vi "子VI-计算分辨率后的值.vi"(7 "测量结果":dbl[][](array[numeric]), 9 "图像X向分辨率（mm/像素）":dbl, 10 "图像Y向分辨率（mm/像素）":dbl) -> (1 "初始化的数组":dbl[][](array[numeric]))   [LabVIEW 2018]
panel:
  out "测量结果 2":dbl[](array[numeric])
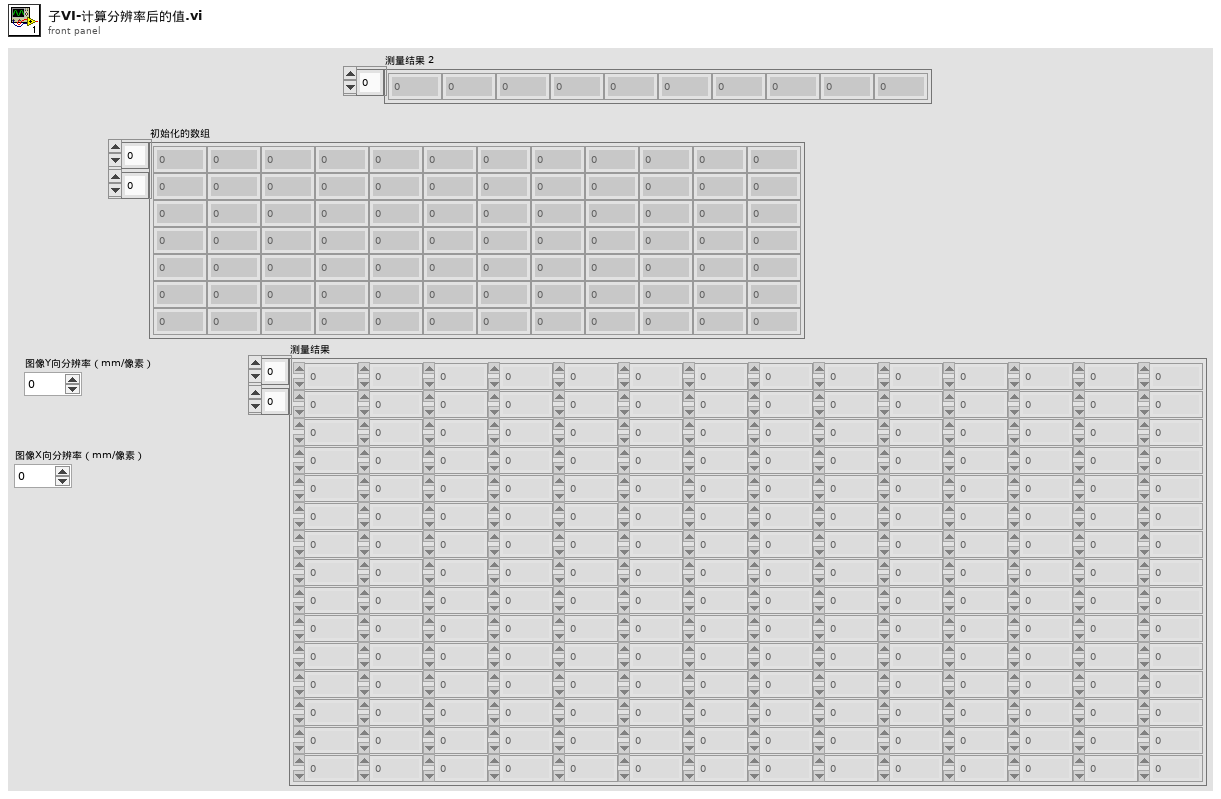
[diagram p1: front panel]
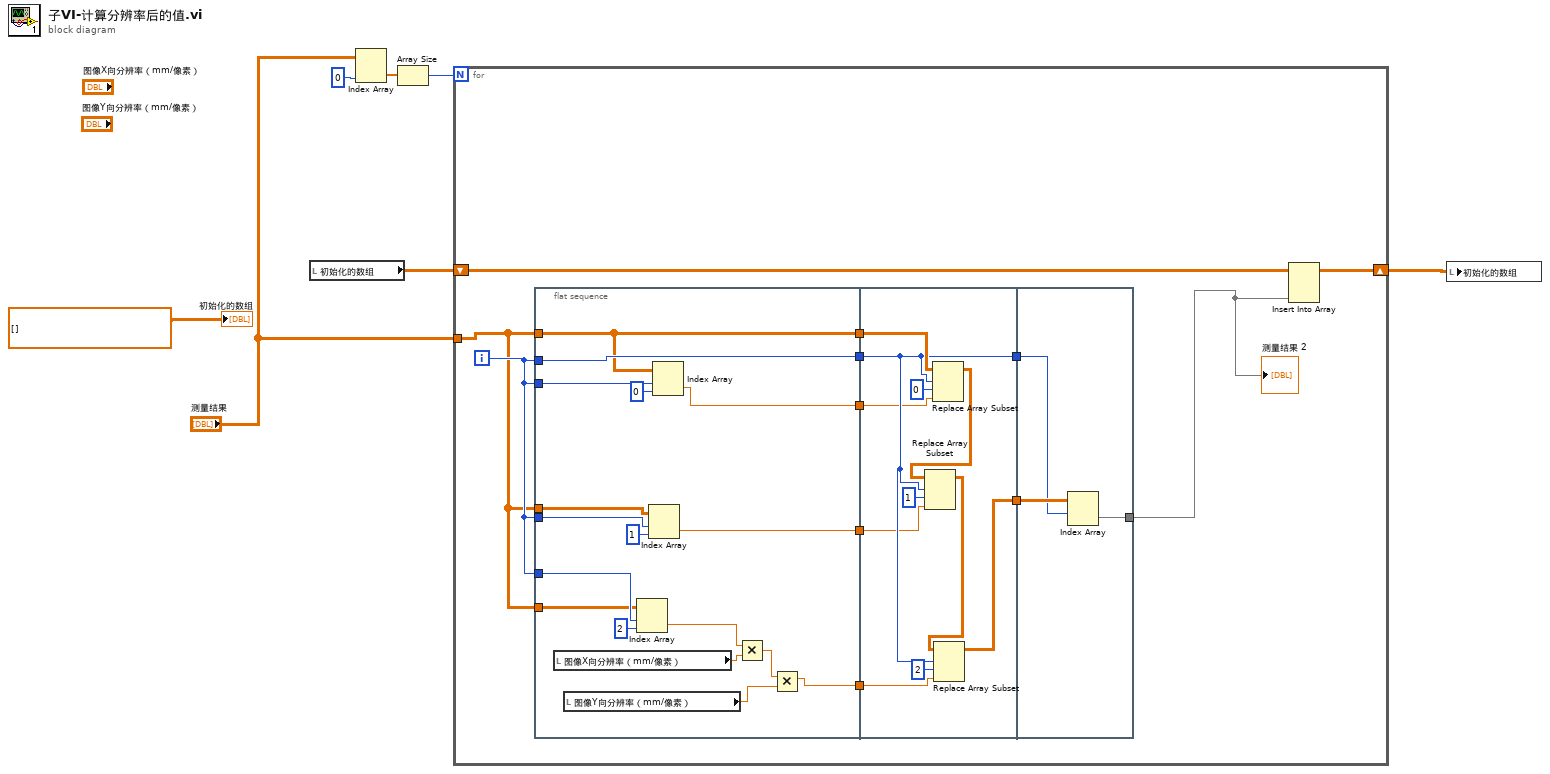
[diagram p0: block diagram]
diagram:
  n1 = local read "初始化的数组"() -> (w2:dbl[][])
  n2 = Index Array(array="测量结果", index (col)=0 ("禁用的索引 (列)")) -> (element=w5:dbl[])  [unwired: 1 in]
  n3 = Array Size(array=w5) -> (size(s)=w6:i32)
  n4 = for {
    N: w6 -> [_]
    tunnel: "测量结果" -> [w11]
    shift-right: [w15] -> w1
    shift-left: w2 -> [w16]
    i -> [w12]
    n5 = flat-sequence {
      tunnel: w11 -> [w32]
      tunnel: w12 -> [w36]
      tunnel: [w32] -> w19
      tunnel: w12 -> [w34]
      tunnel: [w34] -> w18
      tunnel: w12 -> [w31]
      tunnel: w12 -> [w29]
      tunnel: w11 -> [w28]
      tunnel: w11 -> [w27]
      tunnel: [w22] -> w10
      tunnel: [w21] -> w9
      tunnel: [w20] -> w8
      tunnel: w19 -> [w45]
      tunnel: w18 -> [w41]
      tunnel: [w41] -> w17
      tunnel: [w39] -> w14
      tunnel: w10 -> [w42]
      tunnel: w9 -> [w38]
      tunnel: w8 -> [w37]
      tunnel: w17 -> [w49]
      tunnel: w14 -> [w50]
      tunnel: [w48] -> w13
      frame #0 {
        n6 = local read "图像X向分辨率（mm/像素）"() -> (w25:dbl)
        n7 = local read "图像Y向分辨率（mm/像素）"() -> (w23:dbl)
        n8 = Index Array(array=w28, index (row)=w29, index (col)=2 ("禁用的索引 (列)")) -> (element=w26:dbl)
        n9 = Index Array(array=w27, index (row)=w31, index (col)=1 ("禁用的索引 (列)")) -> (element=w20:dbl)
        n10 = Index Array(array=w32, index (row)=w36, index (col)=0 ("禁用的索引 (列)")) -> (element=w21:dbl)
        n11 = Multiply(x=w26, y=w25) -> (x*y=w24:dbl)
        n12 = Multiply(x=w24, y=w23) -> (x*y=w22:dbl)
      }
      frame #1 {
        n13 = Replace Array Subset(array=w45, new element=w38, index (row)=w41, index (col)=0 ("禁用的索引 (列)")) -> (w44:dbl[][])
        n14 = Replace Array Subset(array=w44, new element=w37, index (row)=w41, index (col)=1 ("禁用的索引 (列)")) -> (w40:dbl[][])
        n15 = Replace Array Subset(array=w40, new element=w42, index (row)=w41, index (col)=2 ("禁用的索引 (列)")) -> (w39:dbl[][])
      }
      frame #2 {
        n16 = Index Array(array=w50, index (row)=w49) -> (element=w48:dbl[])  [unwired: 1 in]
      }
    }
    n17 = Insert Into Array(array=w16, new element=w13) -> (w15:dbl[][])  [unwired: 2 in]
    "测量结果 2" <- w13
  }
  n18 = local write "初始化的数组"(w1) -> ()
  "初始化的数组" <- dbl[][] [] ("初始化的数组")
